vi "ScriptClasses.vi"(0 "reference in":refnum<class "Executer.lvclass">, 1 "Filepath":path, 3 "Scripting":refnum<class "Scripting.lvclass">, 5 "error in (no error)":errorcluster) -> (14 "reference out":refnum<class "Executer.lvclass">, 19 "error out":errorcluster)   [LabVIEW 2018, in "Executer.lvclass"]
uses:
  Executer.lvclass
  Scripting/Scripting_class/Scripting.lvclass
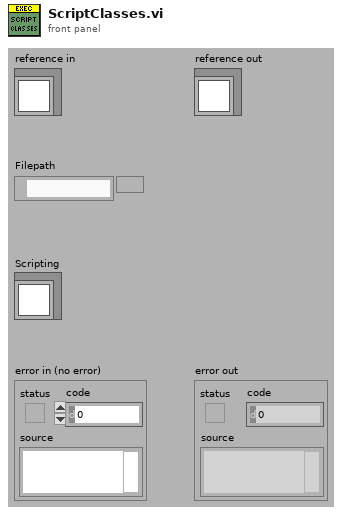
[diagram p1: front panel]
types:
  T1 = typedef "Executer.lvclass/ObjectAttributes.ctl" = cluster{"Executions":T2[]}
  T2 = typedef "Executer.lvclass/ClassExecutionInfo.ctl" = cluster{"Class":refnum<class>, "ClassName":string, "VIExecutionInfo":T3[]}
  T3 = typedef "Executer.lvclass/MethodExecutionInfo.ctl" = cluster{"viRef":refnum<vi>, "MethodName":string, "ControlIndices":i32[], "ClassInIndex":i32, "IndicatorIndices":i32[], "ErrorOutIndex":i32, "ControlTypes":variant[]}
  T4 = typedef "Executer.lvclass/ClassDescription.ctl" = cluster{"ClassName":string, "ClassDescription":string, "MethodDescriptions":T5[]}
  T5 = typedef "Executer.lvclass/MethodDescription.ctl" = cluster{"MethodName":string, "VIDescription":string, "ControlDesciptions":string[], "IndicatorDesciptions":string[], "ControlTypes":variant[], "IndicatorTypes":variant[]}
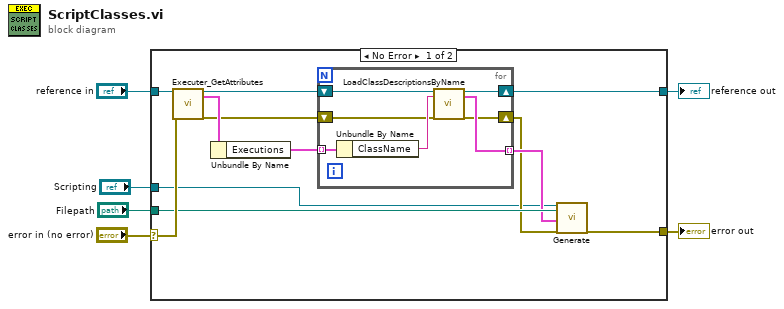
[diagram p0: block diagram]
diagram:
  n1 = case shown="No Error" "error in (no error)" {
    selector: "error in (no error)" -> [w15 w27]
    tunnel: [w17 w27] -> w5
    tunnel: [w11 w26] -> w3
    tunnel: "reference in" -> [w16 w26]
    tunnel: "Filepath" -> [w14 _]
    tunnel: "Scripting" -> [w7 _]
    frame No Error {
      n2 = call "Executer_GetAttributes.vi"("reference in"=w16, "error in (no error)"=w15) -> ("reference out"=w12:refnum<class "Executer.lvclass">, "Data"=w18:T1, "error out"=w8:errorcluster)  [unwired: 14 in, 1 out]
      n3 = Unbundle By Name(w18) -> ("Executions"=w13:T2[])
      n4 = for {
        tunnel: w13 -> [w25] mode=indexing
        shift-right: [w23] -> w11
        shift-left: w12 -> [w24]
        shift-right: [w19] -> w9
        shift-left: w8 -> [w21]
        tunnel: [w20] -> w10 mode=indexing
        n5 = Unbundle By Name(w25) -> ("ClassName"=w22:string)
        n6 = call "LoadClassDescriptionsByName.vi"("Executer in"=w24, "Class in"=w22, "error in (no error)"=w21) -> ("Executer out"=w23:refnum<class "Executer.lvclass">, "ClassDescription"=w20:T4, "error out"=w19:errorcluster)  [unwired: 14 in]
      }
      n7 = call-dynamic "Generate.vi"("reference in"=w7, "Path"=w14, "Classes"=w10, "error in (no error)"=w9) -> ("error out"=w17:errorcluster)  [unwired: 14 in, 1 out]
    }
    frame Error {
    }
  }
  "error out" <- w5
  "reference out" <- w3
